vi "createElement.vi"(6 "firstItem? (F)":bool, 8 "error in (no error)":errorcluster, 9 "prevObjRef":refnum<vi>, 10 "clusterInfo.reference":refnum<vi>, 11 "Element in":refnum<class "Element.lvclass">) -> (0 "error out":errorcluster, 3 "Element out":refnum<class "Element.lvclass">)   [LabVIEW 2016, in "Element.lvclass"]
uses:
  Element.lvclass
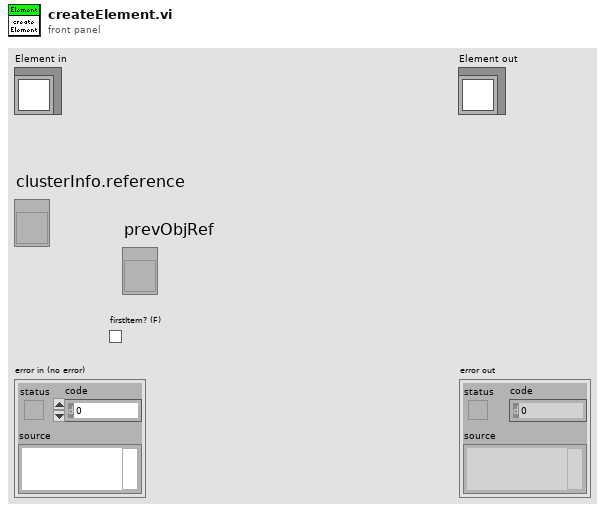
[diagram p1: front panel]
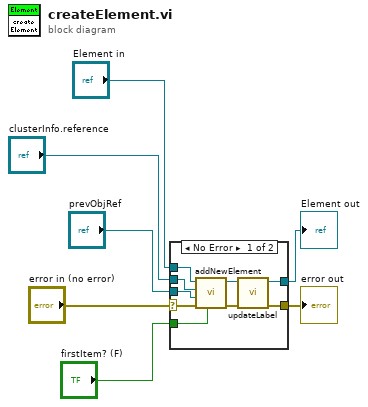
[diagram p0: block diagram]
diagram:
  n1 = case shown="No Error" "error in (no error)" {
    selector: "error in (no error)" -> [w15 w18]
    tunnel: [w8 w18] -> w6
    tunnel: [w10 w17] -> w4
    tunnel: "Element in" -> [w16 w17]
    tunnel: "clusterInfo.reference" -> [w14 _]
    tunnel: "prevObjRef" -> [w13 _]
    tunnel: "firstItem? (F)" -> [w12 _]
    frame No Error {
      n2 = call-dynamic "addNewElement.vi"("firstItem? (F)"=w12, "error in (no error)"=w15, "prevObjRef"=w13, "clusterInfo.reference"=w14, "Element in"=w16) -> ("error out"=w9:errorcluster, "Element out"=w11:refnum<class "Element.lvclass">)  [unwired: 5 in]
      n3 = call "updateLabel.vi"("error in (no error)"=w9, "Element in"=w11) -> ("error out"=w8:errorcluster, "Element out"=w10:refnum<class "Element.lvclass">)  [unwired: 8 in]
    }
    frame Error {
    }
  }
  "error out" <- w6
  "Element out" <- w4
